vi "pcap open dead.vi"(6 "snaplen(65536)":u16=65535, 8 "error in":errorcluster) -> (0 "error out":errorcluster, 3 "pcap_t":u64)   [LabVIEW 2020, in "libpcaplv.lvlib"]
uses:
  libpcaplv.lvlib
  <vilib>/Utility/sysdir.llb/Get System Directory.vi
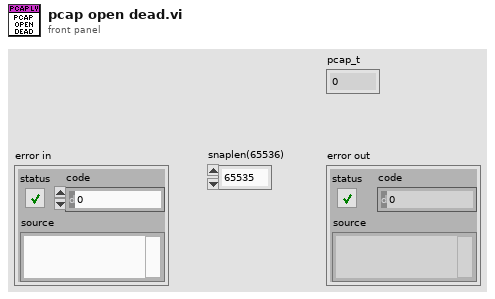
[diagram p1: front panel]
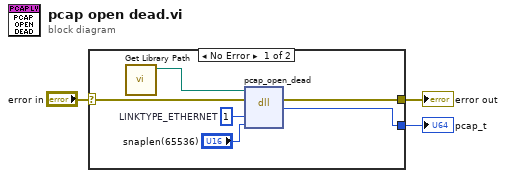
[diagram p0: block diagram]
diagram:
  n1 = case shown="No Error" "error in" {
    selector: "error in" -> [w7 w10]
    tunnel: [w6 _] -> w2
    tunnel: [w5 w10] -> w1
    frame No Error {
      w9 = 1  # LINKTYPE_ETHERNET
      n2 = call "Get Library Path.vi"() -> ("library path"=w4:path)  [unwired: 11 in]
      n3 = dll-call lib="libpcap1.*" fn="pcap_open_dead"(path in=w4, error in=w7, "linktype"=w9, "snaplen"="snaplen(65536)") -> (error out=w5:errorcluster, "pcap_t"=w6:u64)  [unwired: 3 in, 1 out]
    }
    frame Error {
    }
  }
  "pcap_t" <- w2
  "error out" <- w1
